vi "模块1串口初始化.vi"() -> ()   [LabVIEW 2016]
uses:
  <vilib>/Instr/_visa.llb/VISA Configure Serial Port (Instr).vi
panel:
  out "真":bool
  out "布尔 4":bool
  out "布尔 3":bool
  out "布尔 2":bool
  out "布尔":bool
  out "模块四":bool
  out "模块三":bool
  out "模块二":bool
  out "模块一":bool
  out "读取缓冲区":string
  out "正在初始化":u8(slide) scale=0.0..8.0
  out "子字符串;substring 7":string
  out "子字符串;substring 6":string
  out "子字符串;substring 5":string
  out "D1131连接":string
  out "D5131连接":string
  out "D1701连接":string
  out "D1411连接":string
  in  "VISA resource name":refnum<visa-resource-name>="COM3"
  out "循环次数":i32
  # "模块一通信"
  # "模块一初始化"
  # "模块二通信"
  # "模块二初始化"
  # "模块三通信"
  # "模块三初始化"
  # "模块四通信"
  # "模块四初始化"
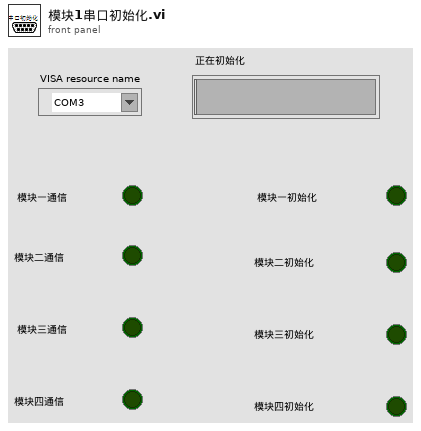
[diagram p1: front panel]
types:
  T1 = enum16{"init", "1", "2", "3", "4", "默认值设置", "初始1", "初始2", "初始3", "初始4"}
  T2 = enum16{"init", "1", "2", "3", "4", "默认值设置", "初始1", "初始2", "初始3"}
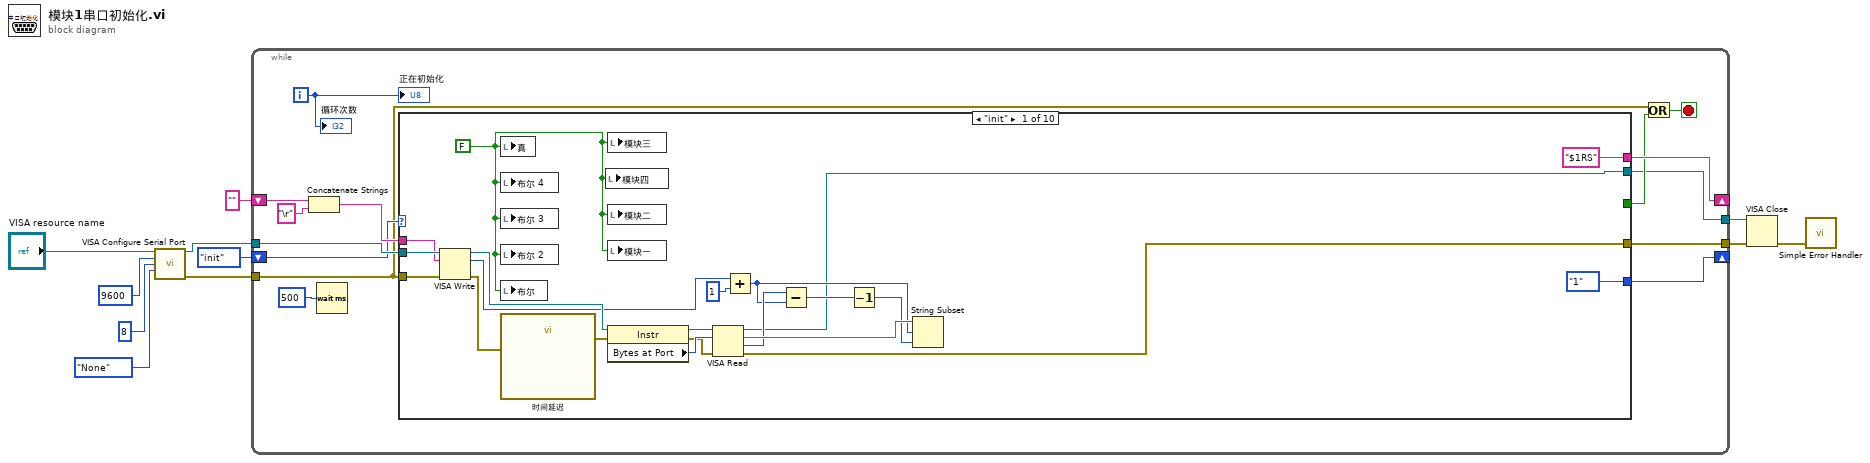
[diagram p0: block diagram]
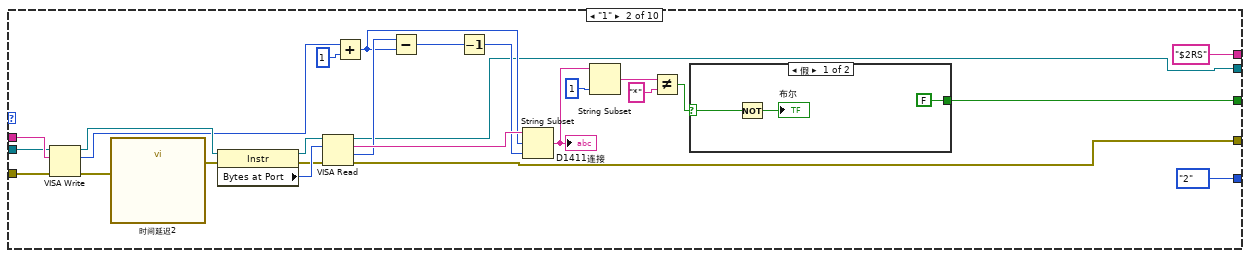
[diagram p2: hidden frame]
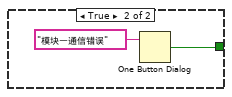
[diagram p3: hidden frame]
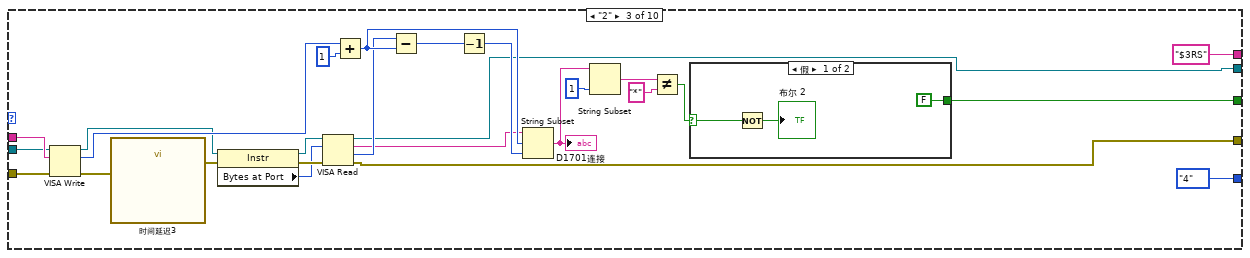
[diagram p4: hidden frame]
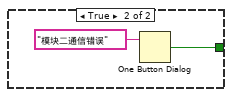
[diagram p5: hidden frame]
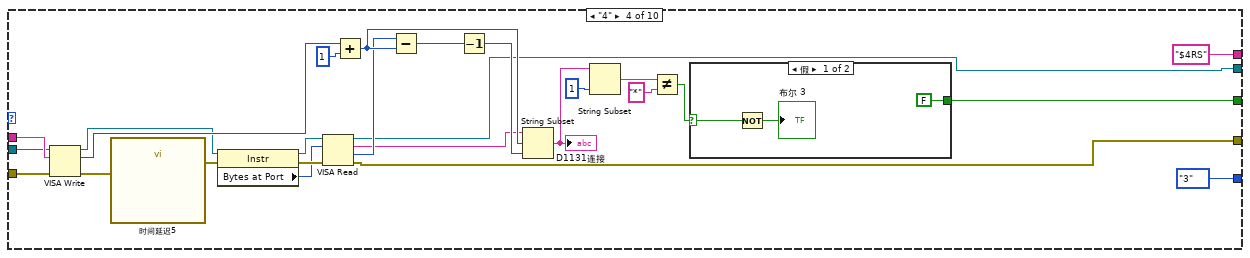
[diagram p6: hidden frame]
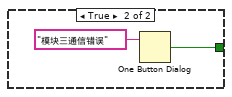
[diagram p7: hidden frame]
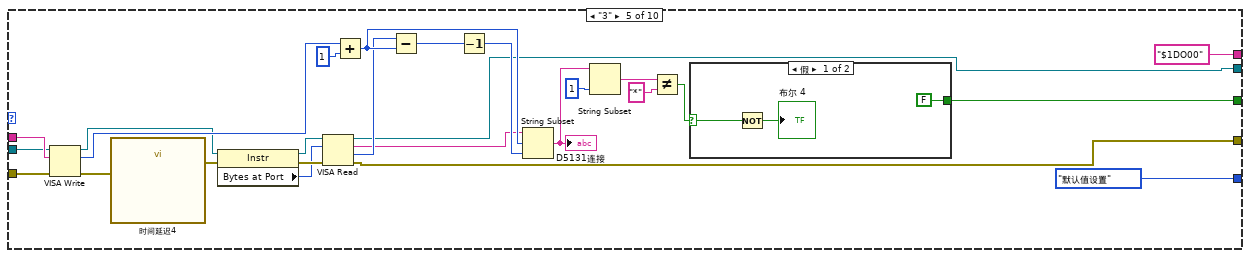
[diagram p8: hidden frame]
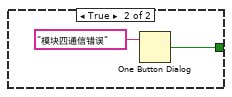
[diagram p9: hidden frame]
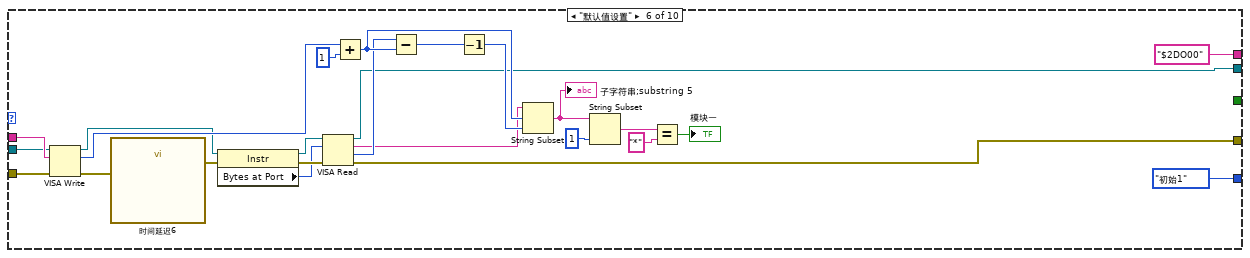
[diagram p10: hidden frame]
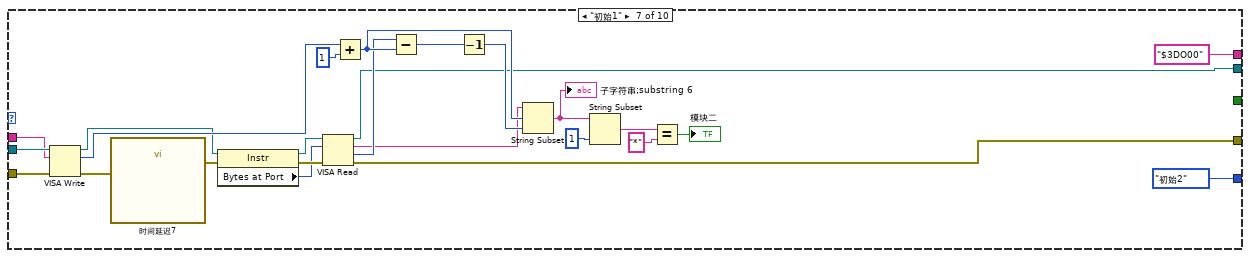
[diagram p11: hidden frame]
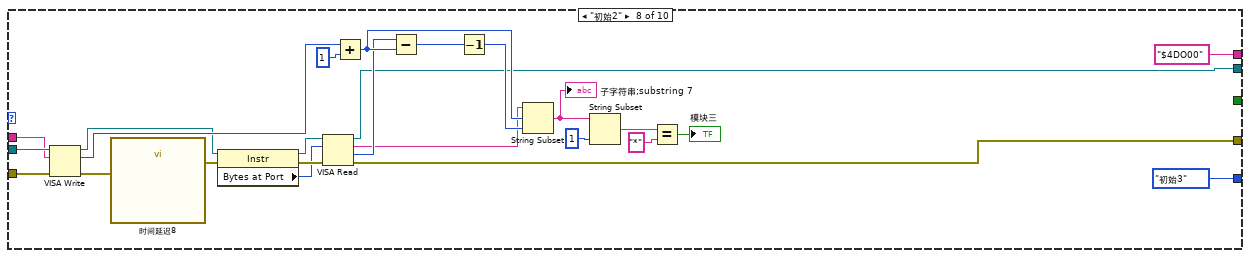
[diagram p12: hidden frame]
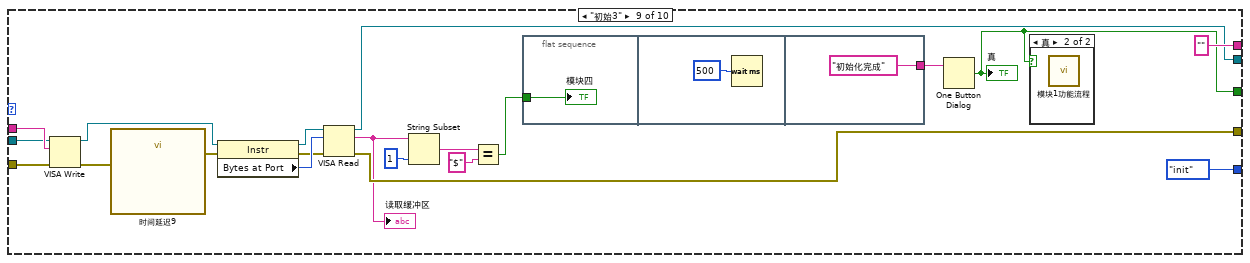
[diagram p13: hidden frame]
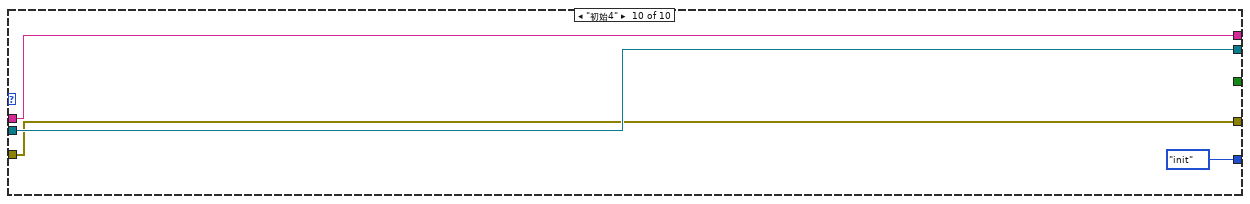
[diagram p15: hidden frame]
diagram:
  n1 = call-poly "VISA Configure Serial Port"("VISA resource name"="VISA resource name", "baud rate (9600)"=9600, "data bits (8)"=8, "parity (0:none)"=enum16{"None", "Odd", "Even", "Mark", "Space"}."None" ("奇偶校验")) -> ("VISA resource name out"=w9:refnum<visa-resource-name>, "error out"=w8:errorcluster)  [unwired: 10 in]
  n2 = while {
    shift-right: [w20] -> _
    shift-left: T1."init" ("枚举") -> [w17]
    shift-right: [w21] -> _
    shift-left: "" -> [w24]
    tunnel: w9 -> [w19]
    tunnel: w8 -> [w12]
    tunnel: [w16] -> w6
    tunnel: [w15] -> w5
    i -> [w14]
    stop <- w13 stop-if-true
    n3 = Concatenate Strings(w24, "\r" ("字符串")) -> (w25:string)
    n4 = Wait (ms)(milliseconds to wait=u32 500 ("等待时间（毫秒）")) -> ()  [unwired: 1 out]
    n5 = case shown="\"init\"" w17 {
      tunnel: [T2."1" ("枚举") T2."2" ("枚举") T2."4" ("枚举") T2."3" ("枚举") T2."默认值设置" ("枚举") T2."初始1" ("枚举") T2."初始2" ("枚举") T2."初始3" ("枚举") T2."init" ("枚举") T2."init" ("枚举")] -> w20
      tunnel: w25 -> [w44 w58 w89 w121 w151 w182 w205 w230 w257 w272]
      tunnel: ["$1RS" ("输入指令") "$2RS" ("输入指令") "$3RS" "$4RS" "$1DO00" "$2DO00" "$3DO00" "$4DO00" "" w272] -> w21
      tunnel: w19 -> [w45 w57 w88 w119 w150 w181 w206 w232 w256 w270]
      tunnel: w12 -> [w43 w56 w87 w120 w149 w180 w207 w231 w255 w269]
      tunnel: [_ w50 w80 w111 w142 _ _ _ w246 _] -> w18
      tunnel: [w28 w53 w85 w116 w147 w177 w202 w227 w253 w270] -> w16
      tunnel: [w27 w54 w84 w115 w146 w176 w201 w226 w252 w269] -> w15
      frame "init" {
        w26 = FALSE ("模块一")
        n6 = VISA Write(VISA resource name=w45, write buffer=w44, error in (no error)=w43) -> (VISA resource name out=w42:refnum<visa-resource-name>, return count=w35:u32, error out=w41:errorcluster)
        n7 = local write "真"(w26) -> ()
        n8 = local write "布尔 4"(w26) -> ()
        n9 = local write "布尔 3"(w26) -> ()
        n10 = local write "布尔 2"(w26) -> ()
        n11 = local write "布尔"(w26) -> ()
        n12 = call "时间延迟"("error in (no error)"=w41) -> ("error out"=w40:errorcluster)  [unwired: 10 in]
        n13 = local write "模块四"(w26) -> ()
        n14 = local write "模块三"(w26) -> ()
        n15 = local write "模块二"(w26) -> ()
        n16 = local write "模块一"(w26) -> ()
        n17 = property class="Instr"(reference=w42, error in=w40) -> (reference out=w39:refnum<visa-resource-name>, error out=w37:errorcluster, "Bytes at Port"=w38:u32)
        n18 = VISA Read(VISA resource name=w39, byte count=w38, error in (no error)=w37) -> (VISA resource name out=w28:refnum<visa-resource-name>, read buffer=w36:string, return count=w33:u32, error out=w27:errorcluster)
        n19 = Add(x=w35, y=u32 1) -> (x+y=w32:u32)
        n20 = Subtract(x=w33, y=w32) -> (x-y=w31:u32)
        n21 = Decrement(x=w31) -> (x-1=w30:u32)
        n22 = String Subset(string=w36, offset (0)=w32, length (rest)=w30) -> ()  [unwired: 1 out]
      }
      frame "1" {
        n23 = VISA Write(VISA resource name=w57, write buffer=w58, error in (no error)=w56) -> (VISA resource name out=w71:refnum<visa-resource-name>, return count=w64:u32, error out=w70:errorcluster)
        n24 = call "时间延迟2"("error in (no error)"=w70) -> ("error out"=w69:errorcluster)  [unwired: 10 in]
        n25 = property class="Instr"(reference=w71, error in=w69) -> (reference out=w68:refnum<visa-resource-name>, error out=w66:errorcluster, "Bytes at Port"=w67:u32)
        n26 = VISA Read(VISA resource name=w68, byte count=w67, error in (no error)=w66) -> (VISA resource name out=w53:refnum<visa-resource-name>, read buffer=w65:string, return count=w62:u32, error out=w54:errorcluster)
        n27 = Add(x=w64, y=u32 1) -> (x+y=w61:u32)
        n28 = Subtract(x=w62, y=w61) -> (x-y=w60:u32)
        n29 = Decrement(x=w60) -> (x-1=w59:u32)
        n30 = String Subset(string=w65, offset (0)=w61, length (rest)=w59) -> (substring=w48:string)
        "D1411连接" <- w48
        n31 = String Subset(string=w48, length (rest)=1 ("长度（剩余）")) -> (substring=w49:string)  [unwired: 1 in]
        n32 = Not Equal?(x=w49, y="*") -> (x != y?=w51:bool)
        n33 = case shown="假" w51 {
          selector: w51 -> [w74 _]
          tunnel: [FALSE w77] -> w50
          frame False {
            n34 = Not(x=w74) -> (.not. x?=→"布尔":bool)
          }
          frame True {
            n35 = One Button Dialog(message="模块一通信错误" ("消息")) -> (true=w77:bool)  [unwired: 1 in]
          }
        }
      }
      frame "2" {
        n36 = VISA Write(VISA resource name=w88, write buffer=w89, error in (no error)=w87) -> (VISA resource name out=w90:refnum<visa-resource-name>, return count=w97:u32, error out=w91:errorcluster)
        n37 = call "时间延迟3"("error in (no error)"=w91) -> ("error out"=w92:errorcluster)  [unwired: 10 in]
        n38 = property class="Instr"(reference=w90, error in=w92) -> (reference out=w93:refnum<visa-resource-name>, error out=w95:errorcluster, "Bytes at Port"=w94:u32)
        n39 = VISA Read(VISA resource name=w93, byte count=w94, error in (no error)=w95) -> (VISA resource name out=w85:refnum<visa-resource-name>, read buffer=w96:string, return count=w99:u32, error out=w84:errorcluster)
        n40 = Add(x=w97, y=u32 1) -> (x+y=w100:u32)
        n41 = Subtract(x=w99, y=w100) -> (x-y=w101:u32)
        n42 = Decrement(x=w101) -> (x-1=w102:u32)
        n43 = String Subset(string=w96, offset (0)=w100, length (rest)=w102) -> (substring=w81:string)
        "D1701连接" <- w81
        n44 = String Subset(string=w81, length (rest)=1 ("长度（剩余）")) -> (substring=w79:string)  [unwired: 1 in]
        n45 = Not Equal?(x=w79, y="*") -> (x != y?=w82:bool)
        n46 = case shown="假" w82 {
          selector: w82 -> [w105 _]
          tunnel: [FALSE w108] -> w80
          frame False {
            n47 = Not(x=w105) -> (.not. x?=→"布尔 2":bool)
          }
          frame True {
            n48 = One Button Dialog(message="模块二通信错误" ("消息")) -> (true=w108:bool)  [unwired: 1 in]
          }
        }
      }
      frame "4" {
        n49 = VISA Write(VISA resource name=w119, write buffer=w121, error in (no error)=w120) -> (VISA resource name out=w122:refnum<visa-resource-name>, return count=w129:u32, error out=w123:errorcluster)
        n50 = call "时间延迟5"("error in (no error)"=w123) -> ("error out"=w124:errorcluster)  [unwired: 10 in]
        n51 = property class="Instr"(reference=w122, error in=w124) -> (reference out=w125:refnum<visa-resource-name>, error out=w127:errorcluster, "Bytes at Port"=w126:u32)
        n52 = VISA Read(VISA resource name=w125, byte count=w126, error in (no error)=w127) -> (VISA resource name out=w116:refnum<visa-resource-name>, read buffer=w128:string, return count=w131:u32, error out=w115:errorcluster)
        n53 = Add(x=w129, y=u32 1) -> (x+y=w132:u32)
        n54 = Subtract(x=w131, y=w132) -> (x-y=w133:u32)
        n55 = Decrement(x=w133) -> (x-1=w134:u32)
        n56 = String Subset(string=w128, offset (0)=w132, length (rest)=w134) -> (substring=w112:string)
        "D1131连接" <- w112
        n57 = String Subset(string=w112, length (rest)=1 ("长度（剩余）")) -> (substring=w110:string)  [unwired: 1 in]
        n58 = Not Equal?(x=w110, y="*") -> (x != y?=w113:bool)
        n59 = case shown="假" w113 {
          selector: w113 -> [w136 _]
          tunnel: [FALSE w139] -> w111
          frame False {
            n60 = Not(x=w136) -> (.not. x?=→"布尔 3":bool)
          }
          frame True {
            n61 = One Button Dialog(message="模块三通信错误" ("消息")) -> (true=w139:bool)  [unwired: 1 in]
          }
        }
      }
      frame "3" {
        n62 = VISA Write(VISA resource name=w150, write buffer=w151, error in (no error)=w149) -> (VISA resource name out=w152:refnum<visa-resource-name>, return count=w159:u32, error out=w153:errorcluster)
        n63 = call "时间延迟4"("error in (no error)"=w153) -> ("error out"=w154:errorcluster)  [unwired: 10 in]
        n64 = property class="Instr"(reference=w152, error in=w154) -> (reference out=w155:refnum<visa-resource-name>, error out=w157:errorcluster, "Bytes at Port"=w156:u32)
        n65 = VISA Read(VISA resource name=w155, byte count=w156, error in (no error)=w157) -> (VISA resource name out=w147:refnum<visa-resource-name>, read buffer=w158:string, return count=w161:u32, error out=w146:errorcluster)
        n66 = Add(x=w159, y=u32 1) -> (x+y=w162:u32)
        n67 = Subtract(x=w161, y=w162) -> (x-y=w163:u32)
        n68 = Decrement(x=w163) -> (x-1=w164:u32)
        n69 = String Subset(string=w158, offset (0)=w162, length (rest)=w164) -> (substring=w143:string)
        "D5131连接" <- w143
        n70 = String Subset(string=w143, length (rest)=1 ("长度（剩余）")) -> (substring=w141:string)  [unwired: 1 in]
        n71 = Not Equal?(x=w141, y="*") -> (x != y?=w144:bool)
        n72 = case shown="假" w144 {
          selector: w144 -> [w167 _]
          tunnel: [FALSE w170] -> w142
          frame False {
            n73 = Not(x=w167) -> (.not. x?=→"布尔 4":bool)
          }
          frame True {
            n74 = One Button Dialog(message="模块四通信错误" ("消息")) -> (true=w170:bool)  [unwired: 1 in]
          }
        }
      }
      frame "默认值设置" {
        n75 = VISA Write(VISA resource name=w181, write buffer=w182, error in (no error)=w180) -> (VISA resource name out=w183:refnum<visa-resource-name>, return count=w190:u32, error out=w184:errorcluster)
        n76 = call "时间延迟6"("error in (no error)"=w184) -> ("error out"=w185:errorcluster)  [unwired: 10 in]
        n77 = property class="Instr"(reference=w183, error in=w185) -> (reference out=w186:refnum<visa-resource-name>, error out=w188:errorcluster, "Bytes at Port"=w187:u32)
        n78 = VISA Read(VISA resource name=w186, byte count=w187, error in (no error)=w188) -> (VISA resource name out=w177:refnum<visa-resource-name>, read buffer=w189:string, return count=w192:u32, error out=w176:errorcluster)
        n79 = Add(x=w190, y=u32 1) -> (x+y=w193:u32)
        n80 = Subtract(x=w192, y=w193) -> (x-y=w194:u32)
        n81 = Decrement(x=w194) -> (x-1=w195:u32)
        n82 = String Subset(string=w189, offset (0)=w193, length (rest)=w195) -> (substring=w175:string)
        "子字符串;substring 5" <- w175
        n83 = String Subset(string=w175, length (rest)=1 ("长度（剩余）")) -> (substring=w172:string)  [unwired: 1 in]
        n84 = Equal?(x=w172, y="*") -> (x = y?=→"模块一":bool)
      }
      frame "初始1" {
        n85 = VISA Write(VISA resource name=w206, write buffer=w205, error in (no error)=w207) -> (VISA resource name out=w208:refnum<visa-resource-name>, return count=w215:u32, error out=w209:errorcluster)
        n86 = call "时间延迟7"("error in (no error)"=w209) -> ("error out"=w210:errorcluster)  [unwired: 10 in]
        n87 = property class="Instr"(reference=w208, error in=w210) -> (reference out=w211:refnum<visa-resource-name>, error out=w213:errorcluster, "Bytes at Port"=w212:u32)
        n88 = VISA Read(VISA resource name=w211, byte count=w212, error in (no error)=w213) -> (VISA resource name out=w202:refnum<visa-resource-name>, read buffer=w214:string, return count=w217:u32, error out=w201:errorcluster)
        n89 = Add(x=w215, y=u32 1) -> (x+y=w218:u32)
        n90 = Subtract(x=w217, y=w218) -> (x-y=w219:u32)
        n91 = Decrement(x=w219) -> (x-1=w220:u32)
        n92 = String Subset(string=w214, offset (0)=w218, length (rest)=w220) -> (substring=w200:string)
        "子字符串;substring 6" <- w200
        n93 = String Subset(string=w200, length (rest)=1 ("长度（剩余）")) -> (substring=w197:string)  [unwired: 1 in]
        n94 = Equal?(x=w197, y="*") -> (x = y?=→"模块二":bool)
      }
      frame "初始2" {
        n95 = VISA Write(VISA resource name=w232, write buffer=w230, error in (no error)=w231) -> (VISA resource name out=w233:refnum<visa-resource-name>, return count=w240:u32, error out=w234:errorcluster)
        n96 = call "时间延迟8"("error in (no error)"=w234) -> ("error out"=w235:errorcluster)  [unwired: 10 in]
        n97 = property class="Instr"(reference=w233, error in=w235) -> (reference out=w236:refnum<visa-resource-name>, error out=w238:errorcluster, "Bytes at Port"=w237:u32)
        n98 = VISA Read(VISA resource name=w236, byte count=w237, error in (no error)=w238) -> (VISA resource name out=w227:refnum<visa-resource-name>, read buffer=w239:string, return count=w242:u32, error out=w226:errorcluster)
        n99 = Add(x=w240, y=u32 1) -> (x+y=w243:u32)
        n100 = Subtract(x=w242, y=w243) -> (x-y=w244:u32)
        n101 = Decrement(x=w244) -> (x-1=w245:u32)
        n102 = String Subset(string=w239, offset (0)=w243, length (rest)=w245) -> (substring=w224:string)
        "子字符串;substring 7" <- w224
        n103 = String Subset(string=w224, length (rest)=1 ("长度（剩余）")) -> (substring=w222:string)  [unwired: 1 in]
        n104 = Equal?(x=w222, y="*") -> (x = y?=→"模块三":bool)
      }
      frame "初始3" {
        n105 = VISA Write(VISA resource name=w256, write buffer=w257, error in (no error)=w255) -> (VISA resource name out=w263:refnum<visa-resource-name>, error out=w262:errorcluster)  [unwired: 1 out]
        n106 = call "时间延迟9"("error in (no error)"=w262) -> ("error out"=w261:errorcluster)  [unwired: 10 in]
        n107 = property class="Instr"(reference=w263, error in=w261) -> (reference out=w260:refnum<visa-resource-name>, error out=w258:errorcluster, "Bytes at Port"=w259:u32)
        n108 = VISA Read(VISA resource name=w260, byte count=w259, error in (no error)=w258) -> (VISA resource name out=w253:refnum<visa-resource-name>, read buffer=w250:string, error out=w252:errorcluster)  [unwired: 1 out]
        "读取缓冲区" <- w250
        n109 = String Subset(string=w250, length (rest)=1 ("长度（剩余）")) -> (substring=w248:string)  [unwired: 1 in]
        n110 = Equal?(x=w248, y="$") -> (x = y?=w249:bool)
        n111 = flat-sequence {
          tunnel: w249 -> [w266]
          tunnel: ["初始化完成" ("消息")] -> w265
          frame #0 {
            "模块四" <- w266
          }
          frame #1 {
            n112 = Wait (ms)(milliseconds to wait=u32 500 ("等待时间（毫秒）")) -> ()  [unwired: 1 out]
          }
          frame #2 {
          }
        }
        n113 = One Button Dialog(message=w265) -> (true=w246:bool)  [unwired: 1 in]
        "真" <- w246
        n114 = case shown="真" w246 {
          frame False {
          }
          frame True {
            n115 = call "模块1功能流程.vi"() -> ()  [unwired: 12 in]
          }
        }
      }
      frame "初始4" {
      }
    }
    n116 = Or(x=w12, y=w18) -> (x .or. y?=w13:bool)
    "循环次数" <- w14
    "正在初始化" <- w14
  }
  n117 = VISA Close(VISA resource name=w6, error in (no error)=w5) -> (error out=w1:errorcluster)
  n118 = call <vilib>:"Simple Error Handler.vi"("error in (no error)"=w1) -> ()  [unwired: 4 in, 5 out]
